vi "Pockels Cal-Calc multiplier for power.vi"(11 "Pockels Cal table":string[][](array[string])=[["Cal Wavelength", "", "", ""], ["820", "", "", ""], ["Prism 1:", "2039", "", ""], ["Prism 2:", "1953", "", ""], ["Laser power displayed (mW):", "3960", "", ""], ["Pockels bias:", "199", "", ""], ["Zoom:", "12", "", ""], ["Dwell time:", "0.4", "", ""], ["Cal subset indexes", "", "", ""], ["0", "15", "", ""], ["Cal data", "", "", ""], ["Pockels V", "No objective", "Nikon 25X", "Olympus 40X"], ["0", "0", "0", "0"], ["0.1", "2.8", "", ""], ["0.2", "9.8", "", ""], ["0.3", "21.4", "", ""], ["0.4", "37.1", "25.97", "37.1"], ["0.5", "56.1", "", ""], ["0.6", "77.7", "", ""], ["0.7", "101", "", ""], ["0.8", "125", "87.5", "125"], ["0.9", "148", "", ""], ["1", "169", "", ""], ["1.1", "188", "", ""], ["1.2", "204", "142.8", "204"], ["1.3", "215", "", ""], ["1.4", "222", "", ""], ["1.5", "225", "", ""], ["1.6", "222", "155.4", "222"], ["1.7", "214", "", ""], ["1.8", "202", "", ""], ["1.9", "187", "", ""], ["2", "152", "106.4", "152"]]) -> (3 "Multiplier for power after the objective":dbl)   [LabVIEW 2013]
uses:
  Program Files (x86)/National Instruments/LabVIEW 2013/user.lib/_OpenG.lib/array/array.llb/Search 1D Array (String)__ogtk.vi
  Program Files (x86)/National Instruments/LabVIEW 2013/user.lib/_OpenG.lib/array/array.llb/Delete Elements from 1D Array (String)__ogtk.vi
  <vilib>/Analysis/NI_AALBase.lvlib
panel:
  out "Ratio per values pair":dbl[](array[numeric])
  out "Power with \"No Objective\"":string[](array[string])
  out "Power with current objective":string[](array[string])
  out "Row index of objective's cal":i32
  out "Column index of objective's cal":i32
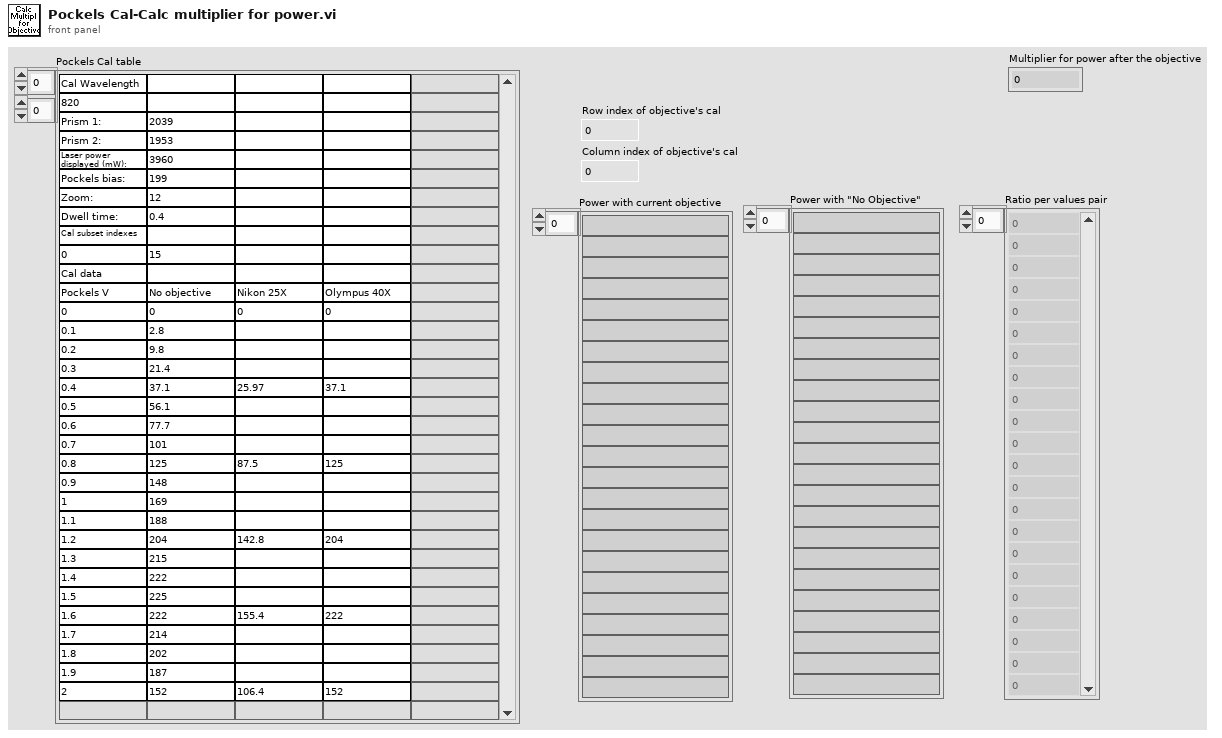
[diagram p1: front panel]
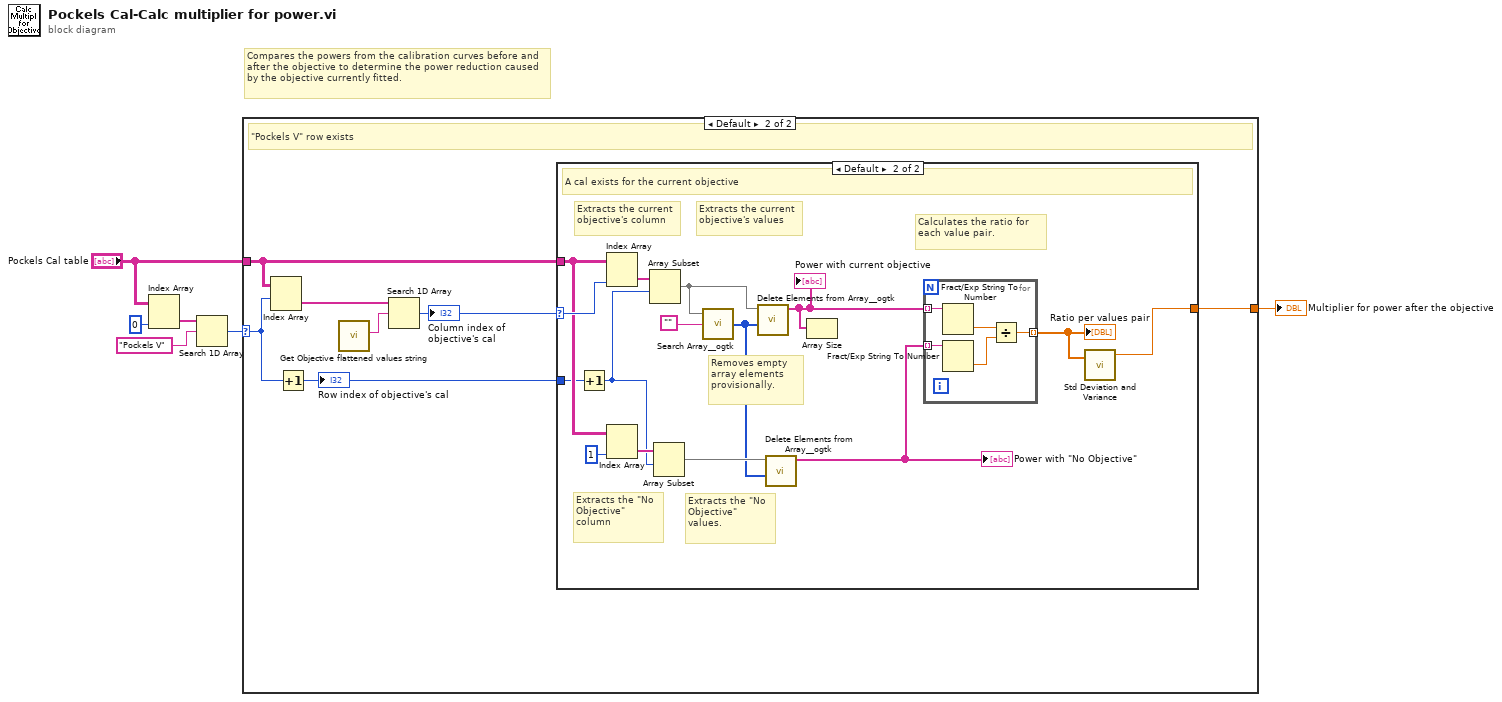
[diagram p0: block diagram]
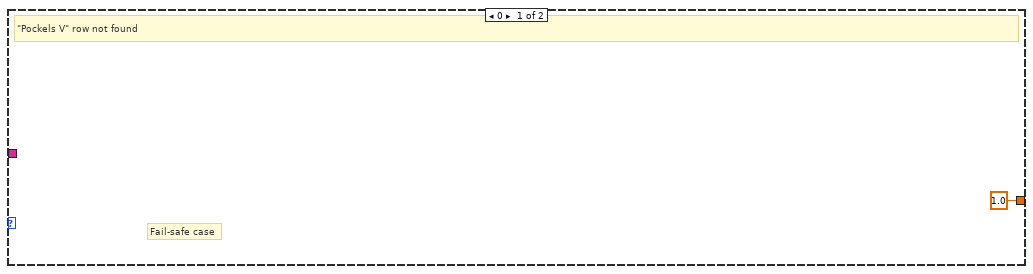
[diagram p2: hidden frame]
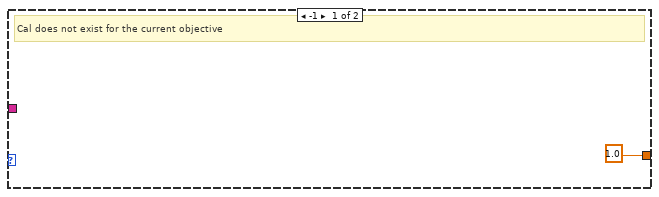
[diagram p3: hidden frame]
diagram:
  # "Compares the powers from the calibration curves before and after the objective to determine the power reduction caused by the objective currently fitted."
  n1 = Index Array(array="Pockels Cal table", index (col)=0 ("disabled index (col)")) -> (element=w4:string[])  [unwired: 1 in]
  n2 = Search 1D Array(1D array=w4, element="Pockels V") -> (index of element=w2:i32)  [unwired: 1 in]
  n3 = case shown="Default" w2 {
    selector: w2 -> [_ w12]
    tunnel: "Pockels Cal table" -> [_ w9]
    tunnel: [1.0 ("Multiplier for power after the objective") w10] -> w1
    frame 0 {
      # "Fail-safe case"
      # "\"Pockels V\" row not found"
    }
    frame Default {
      # "\"Pockels V\" row exists"
      n4 = Index Array(array=w9, index (row)=w12) -> (element=w13:string[])  [unwired: 1 in]
      n5 = Increment(x=w12) -> (x+1=w8:i32)
      "Row index of objective's cal" <- w8
      n6 = call "Get Objective flattened values string.vi"() -> ("Objective.Value"=w14:string)  [unwired: 9 in, 2 out]
      n7 = Search 1D Array(1D array=w13, element=w14) -> (index of element=w11:i32)  [unwired: 1 in]
      "Column index of objective's cal" <- w11
      n8 = case shown="Default" w11 {
        selector: w11 -> [_ w30]
        tunnel: [1.0 ("Multiplier for power after the objective") w20] -> w10
        tunnel: w9 -> [_ w27]
        tunnel: w8 -> [_ w24]
        frame -1 {
          # "Cal does not exist for the current objective"
        }
        frame Default {
          # "Calculates the ratio for each value pair."
          # "Extracts the current objective's values"
          # "Extracts the current objective's column"
          # "Extracts the \"No Objective\" values."
          # "Extracts the \"No Objective\" column"
          # "Removes empty array elements provisionally."
          # "A cal exists for the current objective"
          n9 = Increment(x=w24) -> (x+1=w22:i32)
          n10 = Index Array(array=w27, index (col)=w30) -> (element=w29:string[])  [unwired: 1 in]
          n11 = Index Array(array=w27, index (col)=1 ("disabled index (col)")) -> (element=w25:string[])  [unwired: 1 in]
          n12 = Array Subset(array=w29, index=w22) -> (w19:string[])  [unwired: 1 in]
          n13 = Array Subset(array=w25, index=w22) -> (w18:string[])  [unwired: 1 in]
          n14 = call-poly "Search Array__ogtk.vi"("Array"=w19, "Element Data"="") -> ("Indices of Elements"=w17:i32[])  [unwired: 7 in]
          n15 = call-poly "Delete Elements from Array__ogtk.vi"("indices"=w17, "array"=w19) -> ("array w/ subset deleted"=w23:string[])  [unwired: 8 in, 1 out]
          "Power with current objective" <- w23
          n16 = call-poly "Delete Elements from Array__ogtk.vi"("indices"=w17, "array"=w18) -> ("array w/ subset deleted"=w16:string[])  [unwired: 8 in, 1 out]
          "Power with \"No Objective\"" <- w16
          n17 = Array Size(array=w23) -> ()  [unwired: 1 out]
          n18 = for {
            tunnel: w23 -> [w35] mode=indexing
            tunnel: w16 -> [w34] mode=indexing
            tunnel: [w31] -> w21 mode=indexing
            n19 = Fract/Exp String To Number(string=w35) -> (number=w33:dbl)  [unwired: 3 in, 1 out]
            n20 = Fract/Exp String To Number(string=w34) -> (number=w32:dbl)  [unwired: 3 in, 1 out]
            n21 = Divide(x=w33, y=w32) -> (x/y=w31:dbl)
          }
          "Ratio per values pair" <- w21
          n22 = call <vilib>:"Std Deviation and Variance.vi"("X"=w21) -> ("mean"=w20:dbl)  [unwired: 1 in, 2 out]
        }
      }
    }
  }
  "Multiplier for power after the objective" <- w1
